vi "Ttm-SetPosition.vi"(0 "error in (no error)":errorcluster, 2 "Ttm Name":string="RTC21Summit.RTC.TipTiltMirror.2", 7 "X":dbl, 9 "Y":dbl) -> (3 "error out":errorcluster caption="error in (no error)")   [LabVIEW 2009]
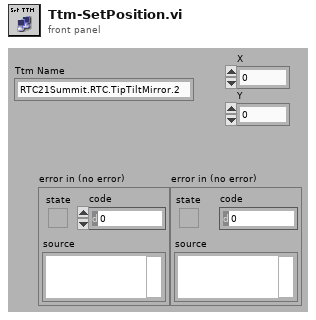
[diagram p1: front panel]
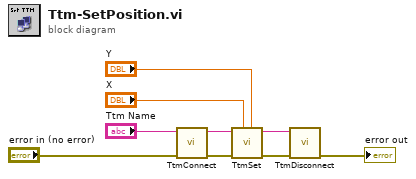
[diagram p0: block diagram]
diagram:
  n1 = call "TtmConnect.vi"("Ttm Name"="Ttm Name", "error in (no error)"="error in (no error)") -> ("Ttm Name out"=w7:string, "error out"=w6:errorcluster)  [unwired: 6 out]
  n2 = call "TtmSet.vi"("Y"="Y", "X"="X", "error in (no error)"=w6, "Ttm Name"=w7) -> ("error out"=w4:errorcluster, "Ttm Name out"=w5:string)  [unwired: 4 out]
  n3 = call "TtmDisconnect.vi"("Ttm Name"=w5, "error in (no error)"=w4) -> ("error out"=→"error out":errorcluster)  [unwired: 7 out]
